vi "Solver.vi"(8 "error in":errorcluster, 11 "Model Data":T1 {"Matricies"."K" format="%#_6e"; "Matricies"."Dout" format="%#_6e"; "Matricies"."Bout" format="%#_6e"; "Matricies"."Aout" format="%#_6e"; "Matricies"."Dint" format="%#_6e"; "Matricies"."Bint" format="%#_6e"; "Matricies"."Aint" format="%#_6e"; "Constants"."Z" format="%^#_6e"}) -> (0 "error out":errorcluster, 3 "Model Data out":T1 {"Matricies"."K" format="%#_6e"; "Matricies"."Dout" format="%#_6e"; "Matricies"."Bout" format="%#_6e"; "Matricies"."Aout" format="%#_6e"; "Matricies"."Dint" format="%#_6e"; "Matricies"."Bint" format="%#_6e"; "Matricies"."Aint" format="%#_6e"; "Constants"."Z" format="%^#_6e"})   [LabVIEW 2022 SP3]
uses:
  Model Data.ctl
  PZT type.ctl
  Piezo_Discs.ctl
  LEM_Params.ctl
  Layer Properties.ctl
  Matricies.ctl
  <vilib>/Utility/error.llb/DialogType.ctl
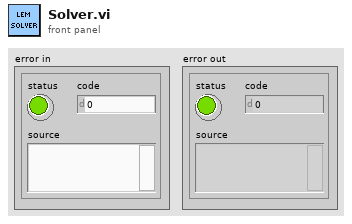
[diagram p1: front panel]
types:
  T1 = typedef "Model Data.ctl" = cluster{"Disc Properties":cluster{"Type":T2, "Disc Model":T3}, "Constants":cluster{"Radius":dbl[], "U(r)":dbl[], "W(r)":dbl[], "Vac":dbl, "P":dbl, "RiRo":dbl, "Area Density (r)":dbl[], "Ro":dbl, "Ri":dbl, "Z":dbl[], "Nr":dbl, "Mr":dbl, "c":dbl[], "AoC":dbl, "BoC":dbl, "AiC":dbl, "BiC":dbl, "f1":dbl, "f2":dbl}, "LEM Parameters":T4, "Layer Properties":T5[], "Matricies":T6}
  T2 = typedef "PZT type.ctl" = enum16{"Bimorph", "Unimorph"}
  T3 = typedef "Piezo_Discs.ctl" = enum16{"FTBD-21T-4.0A1", "PZT-5A (Gallas 1)", "PZT-5A (Gallas 2)", "AB4113B", "Create new disc...", "Load disc from file..."}
  T4 = typedef "LEM_Params.ctl" = cluster{"Displacement Ratio":dbl, "Cd":dbl, "Md":dbl, "xdc":dbl, "fd":dbl, "Sensitivity":dbl, "dA":dbl, "Rd":dbl, "Zeta":dbl, "Phi":dbl}
  T5 = typedef "Layer Properties.ctl" = cluster{"E":dbl, "R":dbl, "rho":dbl, "rhoA":dbl, "v":dbl, "A":dbl, "t":dbl, "d31":dbl, "size":enum16{"Outer", "Inner"}}
  T6 = typedef "Matricies.ctl" = cluster{"Aint":dbl[][], "Bint":dbl[][], "Dint":dbl[][], "Aout":dbl[][], "Bout":dbl[][], "Dout":dbl[][], "b":dbl[], "K":dbl[][]}
  T7 = typedef "DialogType.ctl" = u16
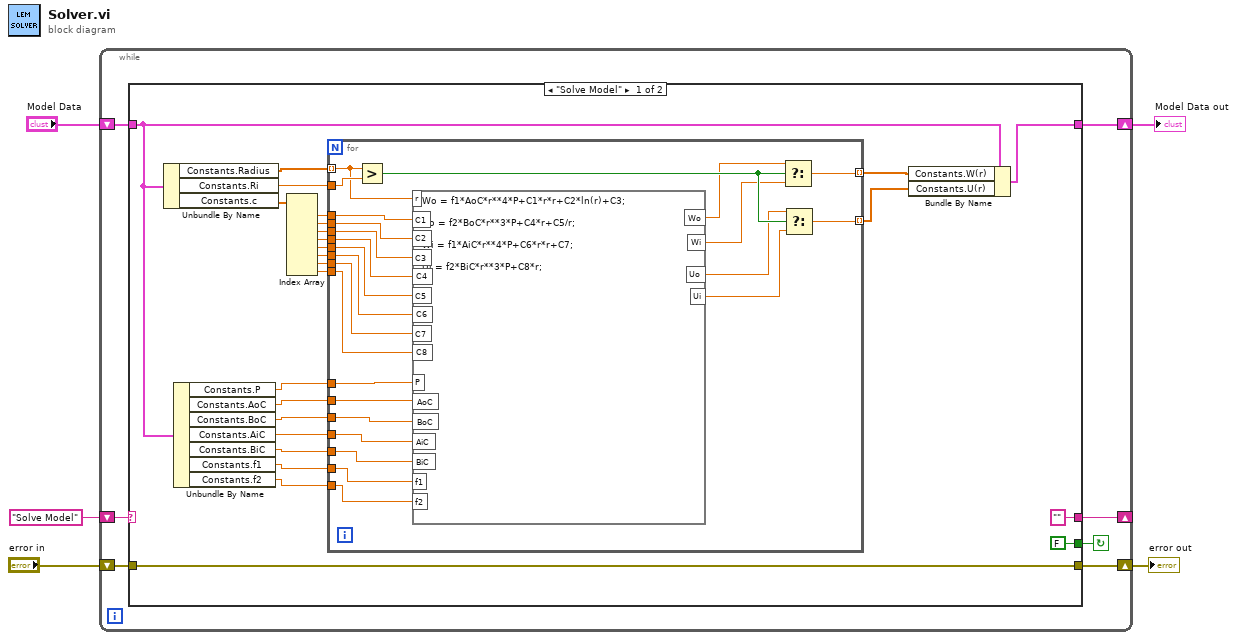
[diagram p0: block diagram]
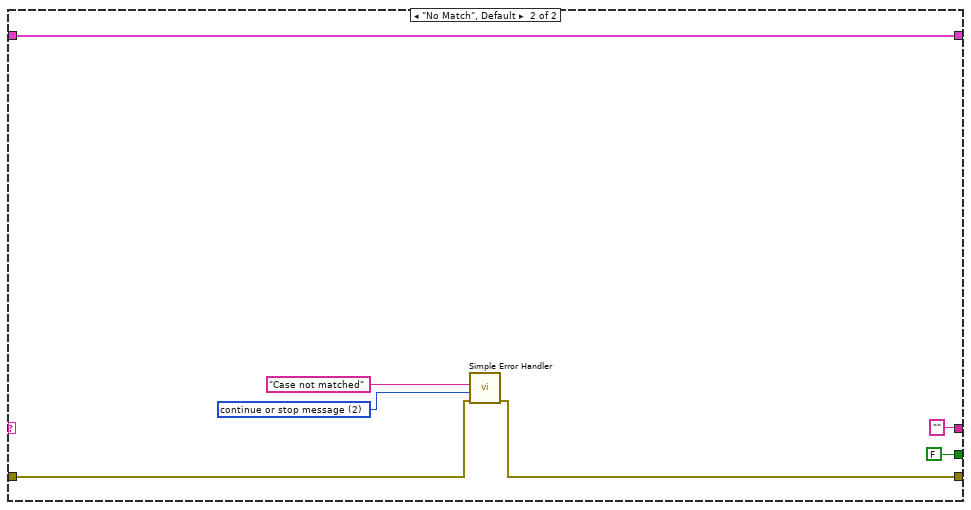
[diagram p2: hidden frame]
diagram:
  n1 = while {
    shift-right: [w9] -> _
    shift-left: "Solve Model" -> [w10]
    shift-right: [w11] -> w1
    shift-left: "Model Data" -> [w8]
    shift-right: [w6] -> w3
    shift-left: "error in" -> [w7]
    stop <- w12 continue-if-true
    n2 = case shown="\"Solve Model\"" w10 {
      tunnel: [FALSE FALSE] -> w12
      tunnel: [w15 w64] -> w11
      tunnel: ["" ""] -> w9
      tunnel: w8 -> [w16 w64]
      tunnel: w7 -> [w37 w63]
      tunnel: [w37 w62] -> w6
      frame "Solve Model" {
        n3 = Unbundle By Name(w16) -> ("Constants.Radius"=w34:dbl[], "Constants.Ri"=w33:dbl, "Constants.c"=w32:dbl[])
        n4 = Unbundle By Name(w16) -> ("Constants.P"=w23:dbl, "Constants.AoC"=w22:dbl, "Constants.BoC"=w21:dbl, "Constants.AiC"=w20:dbl, "Constants.BiC"=w19:dbl, "Constants.f1"=w18:dbl, "Constants.f2"=w17:dbl)
        n5 = Index Array(array=w32) -> (element #1=w31:dbl, element #2=w30:dbl, element #3=w29:dbl, element #4=w28:dbl, element #5=w27:dbl, element #6=w26:dbl, element #7=w25:dbl, element #8=w24:dbl)  [unwired: 8 in]
        n6 = for {
          tunnel: w34 -> [w60] mode=indexing
          tunnel: w33 -> [w61]
          tunnel: w31 -> [w59]
          tunnel: w30 -> [w58]
          tunnel: w29 -> [w57]
          tunnel: w28 -> [w56]
          tunnel: w27 -> [w55]
          tunnel: w26 -> [w54]
          tunnel: w25 -> [w53]
          tunnel: w24 -> [w52]
          tunnel: w23 -> [w51]
          tunnel: w22 -> [w50]
          tunnel: w21 -> [w49]
          tunnel: w20 -> [w45]
          tunnel: w19 -> [w46]
          tunnel: w18 -> [w47]
          tunnel: w17 -> [w48]
          tunnel: [w39] -> w14 mode=indexing
          tunnel: [w38] -> w13 mode=indexing
          n7 = Greater?(x=w60, y=w61) -> (0:w44:bool)
          n8 = formula code="Wo = f1*AoC*r**4*P+C1*r*r+C2*ln(r)+C3;\n\nUo = f2*BoC*r**3*P+C4*r+C5/r;\n\nWi = f1*AiC*r**4*P+C6*r*r+C7;\n\nUi = f2*BiC*r**3*P+C8*r;"("r"=w60, "C1"=w59, "C2"=w58, "C3"=w57, "C4"=w56, "C5"=w55, "C6"=w54, "C7"=w53, "C8"=w52, "P"=w51, "AoC"=w50, "BoC"=w49, "AiC"=w45, "BiC"=w46, "f1"=w47, "f2"=w48) -> ("Wo"=w43:dbl, "Uo"=w41:dbl, "Wi"=w42:dbl, "Ui"=w40:dbl)
          n9 = Select(t=w43, s=w44, f=w42) -> (s? t:f=w39:dbl)
          n10 = Select(t=w41, s=w44, f=w40) -> (s? t:f=w38:dbl)
        }
        n11 = Bundle By Name(cluster=w16, "Constants.W(r)"=w14, "Constants.U(r)"=w13) -> (w15:T1)
      }
      frame "No Match", Default {
        w65 = T7 2 items=["no dialog", "OK message", "continue or stop message", "OK message + warnings", "continue/stop + warnings"] ("type of dialog (OK msg:1)")
        n12 = call <vilib>:"Simple Error Handler.vi"("error source (\" \")"="Case not matched", "type of dialog (OK msg:1)"=w65, "error in (no error)"=w63) -> ("error out"=w62:errorcluster)  [unwired: 2 in, 4 out]
      }
    }
  }
  "error out" <- w3
  "Model Data out" <- w1
